vi "Draw Pod Actual.vi"() -> (3 "Actual Pod Vectors":cluster{dbl[], dbl[]}[](array[cluster]))   [LabVIEW 2020]
uses:
  <vilib>/Rock Robotics/Network Tables/NT Read Numeric Array.vi
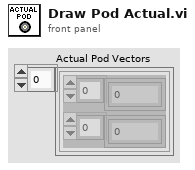
[diagram p1: front panel]
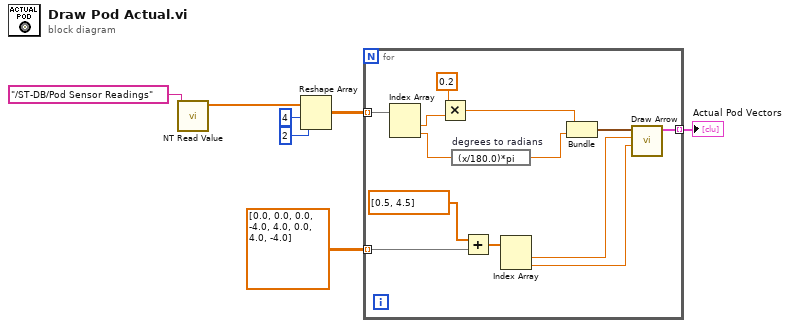
[diagram p0: block diagram]
diagram:
  n1 = call-poly <vilib>:"NT Read Value.vi"("name"="/ST-DB/Pod Sensor Readings") -> ("value"=w6:dbl[])  [unwired: 8 in, 2 out]
  n2 = Reshape Array(w6, 4 ("dimension size"), 2 ("dimension size")) -> (w3:dbl[][])
  n3 = for {
    tunnel: w3 -> [w20] mode=indexing
    tunnel: dbl[][] [[0.0, 0.0], [0.0, -4.0], [4.0, 0.0], [4.0, -4.0]] -> [w18] mode=indexing
    tunnel: [w13] -> w1 mode=indexing
    n4 = Index Array(array=w20) -> (element #1=w12:dbl, element #2=w9:dbl)  [unwired: 2 in]
    n5 = Multiply(x=0.2, y=w12) -> (x*y=w10:dbl)
    n6 = expression code="(x/180.0)*pi" "degrees to radians"(w9) -> (w8:dbl)
    n7 = Add(x=dbl[] [0.5, 4.5], y=w18) -> (x+y=w16:dbl[])
    n8 = Index Array(array=w16) -> (element #1=w15:dbl, element #2=w14:dbl)  [unwired: 2 in]
    n9 = Bundle(w10, "Numeric"=w8) -> (w19:cluster{dbl, "Numeric":dbl})  [unwired: 1 in]
    n10 = call "Draw Arrow.vi"("Start Y"=w14, "Start X"=w15, "Vector"=w19) -> ("Points"=w13:cluster{dbl[], dbl[]})  [unwired: 6 in, 2 out]
  }
  "Actual Pod Vectors" <- w1
